vi "StatusUpdate.vi"(8 "error in (no error)":errorcluster, 9 "Status":string, 10 "ModuleID":i32) -> (0 "error out":errorcluster)   [LabVIEW 2014, in "FlagImpairModule.lvlib"]
uses:
  FlagImpairModule.lvlib
  PublicAPI/Arguments/Broadcasts/clStatUpdate.ctl
  clEventType.ctl
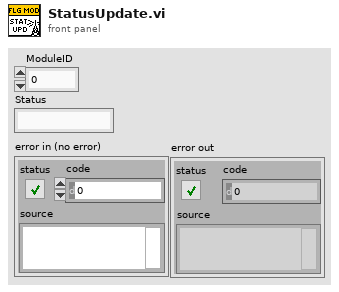
[diagram p1: front panel]
types:
  T1 = typedef "FlagImpairModule.lvlib/clEventType.ctl" = cluster{"ModuleID":i32, "Data":variant}
  T2 = typedef "FlagImpairModule.lvlib/clStatUpdate.ctl" = cluster{"Status":string}
  T3 = typedef "FlagImpairModule.lvlib/clBroadcastEvents.ctl" = cluster{"DidInit":refnum<user-event>, "StatusUpdate":refnum<user-event>, "ErrorReport":refnum<user-event>, "DidStop":refnum<user-event>, "ReadFlagImpairConfig":refnum<user-event>, "ReadPluginINIFilePath":refnum<user-event>, "ReadFlagImpairParams":refnum<user-event>, "ReadTimeArray":refnum<user-event>, "GetFlagImpairment":refnum<user-event>}
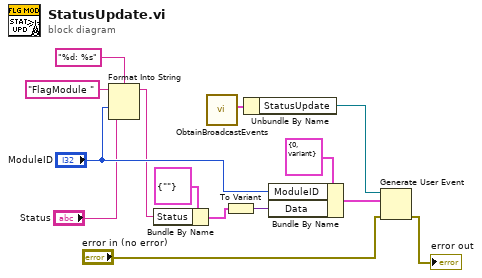
[diagram p0: block diagram]
diagram:
  n1 = Format Into String(format string="%d: %s", initial string="FlagModule ", "ModuleID", "Status") -> (resulting string=w1:string)  [unwired: 1 in, 1 out]
  n2 = Bundle By Name(cluster=T2 {"Status"=""} ("clStatUpdate"), "Status"=w1) -> (w11:T2)
  n3 = call "ObtainBroadcastEvents.vi"() -> ("clBroadcastEvents"=w13:T3)  [unwired: 10 in, 1 out]
  n4 = To Variant(anything=w11) -> (Variant=w9:variant)
  n5 = Unbundle By Name(w13) -> ("StatusUpdate"=w12:refnum<user-event>)
  n6 = Bundle By Name(cluster=T1 {"ModuleID"=0, "Data"=variant} ("clBroadcast"), "ModuleID"="ModuleID", "Data"=w9) -> (w8:T1)
  n7 = Generate User Event(user event=w12, event data cluster=w8, error in="error in (no error)") -> (error out=→"error out":errorcluster)  [unwired: 1 in, 1 out]
